vi "MQTT_Disconnect.vi"(8 "error in (no error)":errorcluster, 11 "connection ID":refnum<k5>) -> (0 "error out":errorcluster)   [LabVIEW 2024, in "MQTT_Functions.lvlib"]
doc: "Disconnects from an MQTT broker server.\n\n© 2015 - daq.io, LLC - Peter Adelhardt"
uses:
  MQTT_Functions.lvlib
  Controls/MessageType.ctl
  Controls/Retain_Flag.ctl
  Controls/QoS.ctl
  Controls/DUP_Flag.ctl
  Controls/Conn_FGV_Cmds.ctl
  Controls/Conn_Stat_FGV_Cmds.ctl
  Controls/Connection_Return_Codes.ctl
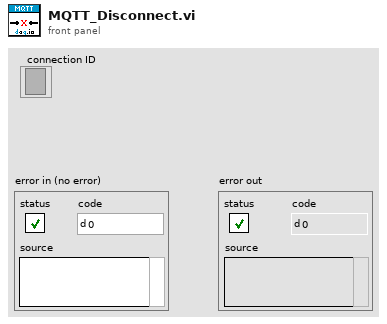
[diagram p1: front panel]
types:
  T1 = typedef "MQTT_Functions.lvlib/DUP_Flag.ctl" = bool
  T2 = typedef "MQTT_Functions.lvlib/QoS.ctl" = enum8{"At most once", "At least once", "Exactly once", "Reserved"}
  T3 = typedef "MQTT_Functions.lvlib/Retain_Flag.ctl" = bool
  T4 = typedef "MQTT_Functions.lvlib/MessageType.ctl" = enum32{"Reserved", "CONNECT", "CONNACK", "PUBLISH", "PUBACK", "PUBREC", "PUBREL", "PUBCOMP", "SUBSCRIBE", "SUBACK", "UNSUBSCRIBE", "UNSUBACK", "PINGREQ", "PINGRESP", "DISCONNECT", "Reserved2"}
  T5 = typedef "MQTT_Functions.lvlib/Conn_FGV_Cmds.ctl" = enum16{"Get", "Set", "Delete"}
  T6 = typedef "MQTT_Functions.lvlib/Connection_Return_Codes.ctl" = enum16{"Connection accepted", "Connection refused: unacceptable protocol version", "Connection refused: identifier rejected", "Connection refused: Server unavailable", "Connection refused: bad user name or password", "Connection refused: not authorized"}
  T7 = typedef "MQTT_Functions.lvlib/Conn_Stat_FGV_Cmds.ctl" = enum16{"Get", "Set"}
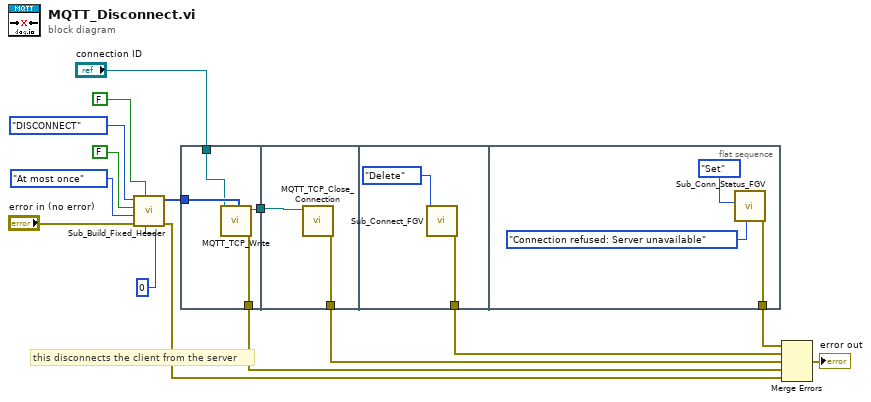
[diagram p0: block diagram]
diagram:
  # "this disconnects the client from the server"
  n1 = call "Sub_Build_Fixed_Header.vi"("Remaining Length"=u32 0, "Retain"=T3 FALSE, "error in (no error)"="error in (no error)", "QoS"=QoS."At most once", "DUP"=T1 FALSE, "MessageType"=MessageType."DISCONNECT") -> ("error out"=w2:errorcluster, "Fixed Header"=w8:u8[])  [unwired: 4 in]
  n2 = flat-sequence {
    tunnel: [w17] -> w9
    tunnel: w8 -> [w19]
    tunnel: "connection ID" -> [w18]
    tunnel: [w16] -> w3
    tunnel: w9 -> [w21]
    tunnel: [w20] -> w4
    tunnel: [w22] -> w5
    tunnel: [w24] -> w6
    frame #0 {
      n3 = call "MQTT_TCP_Write.vi"("data in"=w19, "connection ID"=w18) -> ("error out"=w16:errorcluster, "connection ID out"=w17:refnum<k5>)  [unwired: 7 in, 1 out]
    }
    frame #1 {
      n4 = call "MQTT_TCP_Close_Connection.vi"("connection ID"=w21) -> ("error out"=w20:errorcluster)  [unwired: 9 in, 1 out]
    }
    frame #2 {
      n5 = call "Sub_Connect_FGV.vi"("Command"=Conn_FGV_Cmds."Delete") -> ("error out"=w22:errorcluster)  [unwired: 9 in, 1 out]
    }
    frame #3 {
      n6 = call "Sub_Conn_Status_FGV.vi"("Connection Status in"=Connection_Return_Codes."Connection refused: Server unavailable", "Command"=Conn_Stat_FGV_Cmds."Set") -> ("error out"=w24:errorcluster)  [unwired: 8 in, 1 out]
    }
  }
  n7 = Merge Errors(w6, w5, w4, w3, w2) -> (→"error out":errorcluster)
